vi "BAE5.vi"() -> ()   [LabVIEW 2014]
doc: "BAE5\n\nOpens and reads a file with a navigating directory upon execution. The program then extracts the following values as data: starting, step, and ending temperature, and number of cycles per temperature average, number of points per timed measurement sequence, and timed interval. These values are then displayed accordingly on the front panel.\n\nAlso, based on the last value of the text file, an indicator will light up for one and be dim otherwise.\n\nBeverly Abadines\nPHY 350\nBAE5s"
uses:
  typedefs/temp control params.ctl
  typedefs/time control params.ctl
panel:
  out "time control parameters":T1 {"Measurment time interval" format="%.2e"}
  out "temp control parameters":T2 {"End Temp" format="%.2f"; "Temp Step" format="%.2f"; "Start Temp" format="%.2f"}
  in  "stop":bool
  out "file path used":path
  out "?":bool
  # "Beverly Abadines\nPHY 350\nBAE5"
  # "Initialization File Parser"
  # "Auto Launch Data Viewer at End"
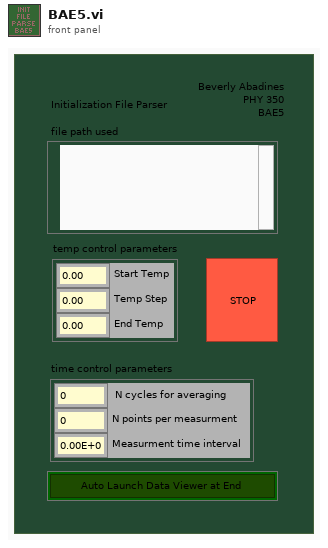
[diagram p1: front panel]
types:
  T1 = typedef "time control params.ctl" = cluster{"N cycles for averaging":i32, "N points per measurment":i32, "Measurment time interval":dbl}
  T2 = typedef "temp control params.ctl" = cluster{"Start Temp":dbl, "Temp Step":dbl, "End Temp":dbl}
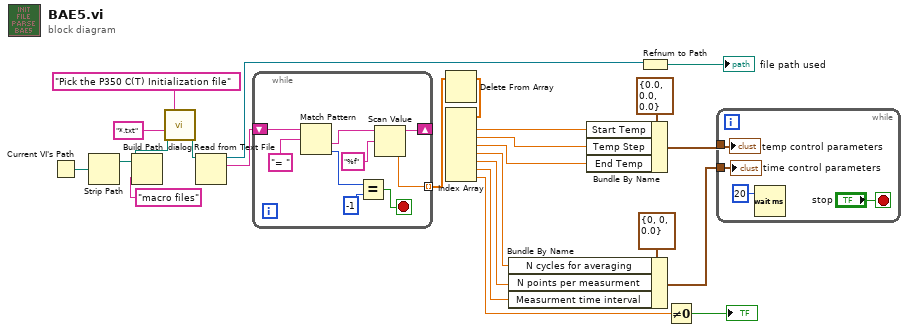
[diagram p0: block diagram]
diagram:
  n1 = Current VI's Path() -> (path=w7:path)
  n2 = Strip Path(path=w7) -> (stripped path=w6:path)  [unwired: 1 out]
  n3 = Build Path(base path=w6, name or relative path="macro files") -> (appended path=w3:path)
  n4 = call "dialog.vi"("start path"=w3, "prompt"="Pick the P350 C(T) Initialization file", "pattern (all files)"="*.txt" ("pattern")) -> ("selected path"=w1:path)  [unwired: 9 in, 3 out]
  n5 = Read from Text File(file (use dialog)=w1) -> (refnum out=w18:refnum<file>, text=w24:string)  [unwired: 3 in, 2 out]
  n6 = while {
    shift-right: [w30] -> _
    shift-left: w24 -> [w33]
    tunnel: [w25] -> w23 mode=indexing
    stop <- w28 stop-if-true
    n7 = Match Pattern(string=w33, regular expression="= " ("in slash mode")) -> (after substring=w29:string, offset past match=w26:i32)  [unwired: 1 in, 2 out]
    n8 = Equal?(x=w26, y=-1) -> (x = y?=w28:bool)
    n9 = Scan Value(string=w29, format string="%f") -> (output string=w30:string, value=w25:dbl)  [unwired: 1 in]
  }
  n10 = Delete From Array(array=w23) -> (array with subset deleted=w22:dbl[])  [unwired: 2 in, 1 out]
  n11 = Index Array(array=w22) -> (element #1=w16:dbl, element #2=w15:dbl, element #3=w14:dbl, element #4=w13:dbl, element #5=w12:dbl, element #6=w11:dbl, element #7=w10:dbl)  [unwired: 7 in]
  n12 = Bundle By Name(cluster=T1 {"N cycles for averaging"=0, "N points per measurment"=0, "Measurment time interval"=0.0} ("time control parameters"), "N cycles for averaging"=w13, "N points per measurment"=w12, "Measurment time interval"=w11) -> (w8:T1)
  n13 = Bundle By Name(cluster=T2 {"Start Temp"=0.0, "Temp Step"=0.0, "End Temp"=0.0} ("temp control parameters"), "Start Temp"=w16, "Temp Step"=w15, "End Temp"=w14) -> (w9:T2)
  n14 = Refnum to Path(1:w18) -> (0:→"file path used":path)
  n15 = Not Equal To 0?(x=w10) -> (x != 0?=→"?":bool)
  n16 = while {
    tunnel: w9 -> [w35]
    tunnel: w8 -> [w34]
    stop <- "stop" stop-if-true
    n17 = Wait (ms)(milliseconds to wait=u32 20) -> ()  [unwired: 1 out]
    "temp control parameters" <- w35
    "time control parameters" <- w34
  }
